vi "Set PPL for This Target.vi"(8 "error in":errorcluster, 10 "path file name":string) -> (0 "error out":errorcluster)   [LabVIEW 2017]
uses:
  PPL Path Info.ctl
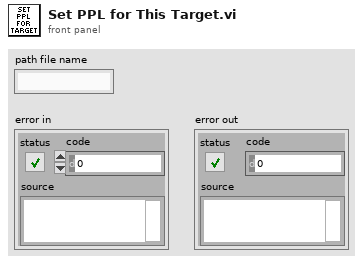
[diagram p1: front panel]
types:
  T1 = typedef "PPL Path Info.ctl" = cluster{"Destination":path, "Sources":cluster{"Linux 32":path, "Linux 64":path, "Win 32":path, "Win 64":path, "Pharlap":path}}
  T2 = cluster{"Destination":string, "Sources":cluster{"Linux 32":string, "Linux 64":string, "Win 32":string, "Win 64":string, "Pharlap":string}}
  T3 = cluster{"Destination":path, "Sources":cluster{"Linux 32":path, "Linux 64":path, "Win 32":path, "Win 64":path, "Pharlap":path}}
  T4 = cluster{"Linux 32":path, "Linux 64":path, "Win 32":path, "Win 64":path, "Pharlap":path}
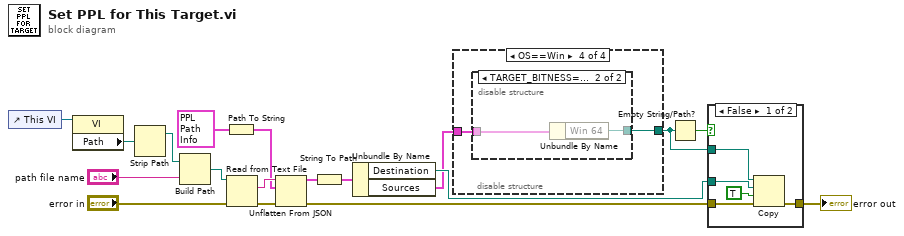
[diagram p0: block diagram]
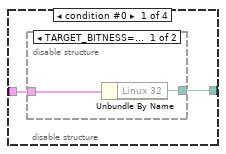
[diagram p3: hidden frame]
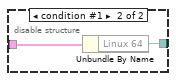
[diagram p4: hidden frame]
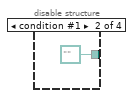
[diagram p5: hidden frame]
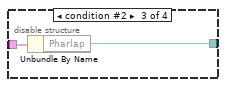
[diagram p6: hidden frame]
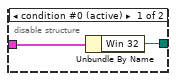
[diagram p7: hidden frame]
diagram:
  n1 = control-ref of="This VI"() -> (w7:refnum<vi>)
  n2 = property class="VI"(reference=w7) -> ("Path"=w3:path)  [unwired: 1 in, 2 out]
  n3 = Strip Path(path=w3) -> (stripped path=w2:path)  [unwired: 1 out]
  n4 = Build Path(base path=w2, name or relative path="path file name") -> (appended path=w6:path)
  n5 = Path To String(path=T1 {"Destination"=path "", "Sources"={"Linux 32"=path "", "Linux 64"=path "", "Win 32"=path "", "Win 64"=path "", "Pharlap"=path ""}} ("PPL Paths")) -> (string=w5:T2)
  n6 = Read from Text File(file (use dialog)=w6, error in="error in") -> (text=w18:string, error out=w11:errorcluster)  [unwired: 2 in, 2 out]
  n7 = Unflatten From JSON(JSON string=w18, type and defaults=w5, error in (no error)=w11) -> (value=w17:T2, error out=w12:errorcluster)  [unwired: 4 in]
  n8 = String To Path(string=w17) -> (path=w16:T3)
  n9 = Unbundle By Name(w16) -> ("Destination"=w14:path, "Sources"=w13:T4)
  n10 = disable-structure shown="OS==Win" {
    disable-tunnel: [w19 path "" ("source path") w26 w28] -> w9
    disable-tunnel: w13 -> [w20 _ w27 w29]
    frame condition #0 {
      n11 = disable-structure shown="TARGET_BITNESS==32, Default" {
        disable-tunnel: w20 -> [w22 w24]
        disable-tunnel: [w21 w23] -> w19
        frame condition #0 (active) {
          n12 = Unbundle By Name(w22) -> ("Linux 32"=w21:path)
        }
        frame condition #1 {
          n13 = Unbundle By Name(w24) -> ("Linux 64"=w23:path)
        }
      }
    }
    frame condition #1 {
    }
    frame condition #2 {
      n14 = Unbundle By Name(w27) -> ("Pharlap"=w26:path)
    }
    frame condition #3 (active) {
      n15 = disable-structure shown="TARGET_BITNESS==64" {
        disable-tunnel: w29 -> [w31 w33]
        disable-tunnel: [w30 w32] -> w28
        frame condition #0 (active) {
          n16 = Unbundle By Name(w31) -> ("Win 32"=w30:path)
        }
        frame condition #1 {
          n17 = Unbundle By Name(w33) -> ("Win 64"=w32:path)
        }
      }
    }
  }
  n18 = Empty String/Path?(string/path=w9) -> (empty?=w8:bool)
  n19 = case shown="False" w8 {
    tunnel: w14 -> [w38 _]
    tunnel: w9 -> [w37 _]
    tunnel: w12 -> [w35 w39]
    tunnel: [w34 w39] -> w10
    frame False {
      n20 = Copy(8:w35, 9:TRUE ("overwrite (F)"), 10:w38, 11:w37) -> (0:w34:errorcluster)  [unwired: 1 in, 2 out]
    }
    frame True {
    }
  }
  "error out" <- w10
